vi "bodyGlobal.vi"() -> ()   [LabVIEW 2013]
uses:
  <vilib>/MakerHub/KinectOne/Private/Type Defs/BodyData.ctl
  <vilib>/MakerHub/KinectOne/Private/Type Defs/ClippedEdges.ctl
  <vilib>/MakerHub/KinectOne/Private/Type Defs/HandLeftConfidence.ctl
  <vilib>/MakerHub/KinectOne/Private/Type Defs/HandLeftState.ctl
  <vilib>/MakerHub/KinectOne/Private/Type Defs/HandRightConfidence.ctl
  <vilib>/MakerHub/KinectOne/Private/Type Defs/HandRightState.ctl
  Microsoft.Kinect
  <vilib>/MakerHub/KinectOne/Private/Type Defs/LeanTrackingState.ctl
  <vilib>/MakerHub/KinectOne/KinectOne.lvlib
panel:
  in  "Body Data":T1[](array[typedef])
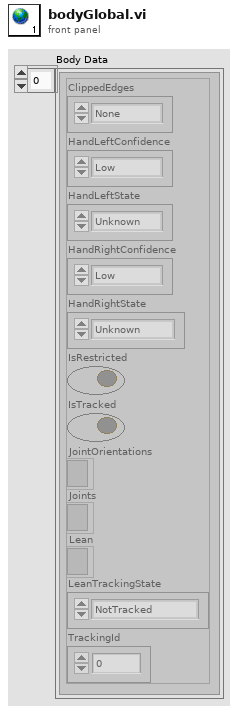
[diagram p1: front panel]
types:
  T1 = typedef "KinectOne.lvlib/BodyData.ctl" = cluster{"ClippedEdges":T2, "HandLeftConfidence":T3, "HandLeftState":T4, "HandRightConfidence":T5, "HandRightState":T6, "IsRestricted":bool, "IsTracked":bool, "JointOrientations":refnum<k24>, "Joints":refnum<k24>, "Lean":refnum<k24>, "LeanTrackingState":T7, "TrackingId":u64}
  T2 = typedef "KinectOne.lvlib/ClippedEdges.ctl" = enum16{"None", "Right", "Left", "Top", "Bottom"}
  T3 = typedef "KinectOne.lvlib/HandLeftConfidence.ctl" = enum16{"Low", "High"}
  T4 = typedef "KinectOne.lvlib/HandLeftState.ctl" = enum16{"Unknown", "NotTracked", "Open", "Closed", "Lasso"}
  T5 = typedef "KinectOne.lvlib/HandRightConfidence.ctl" = enum16{"Low", "High"}
  T6 = typedef "KinectOne.lvlib/HandRightState.ctl" = enum16{"Unknown", "NotTracked", "Open", "Closed", "Lasso"}
  T7 = typedef "KinectOne.lvlib/LeanTrackingState.ctl" = enum16{"NotTracked", "Inferred", "Tracked"}
diagram:
